vi "CRYSet Statistics Run Flag.vi"(0 "Results in":T1 {"Margin" format="%.2f"}, 1 "Data in":T3 {"Z data" items=["dB", "Lin"]; "X data" items=["dB", "Lin"]; "Y data" items=["dB", "Lin"]; "Z dB ref" format="%.1f"; "Z axis" items=["Log", "Lin"]; "X dB ref" format="%.1f"; "X axis" items=["Log", "Lin"]; "Y axis" items=["Log", "Lin"]; "Y dB ref" format="%.1f"; "Curve"."z" format="%.2f"; "Curve"."y" format="%.2f"; "Curve"."x" format="%.2f"}, 5 "Mode":u16(slide), 9 "Dat_State":bool[](array[boolean]), 11 "Res_state":bool[](array[boolean]), 12 "USL":dbl, 13 "LSL":dbl) -> (4 "Run flag":bool, 10 "Message Numbers":i32[](array[numeric]))   [LabVIEW 2013]
uses:
  Typedef Control/CRYData Cluster Array.ctl
  Typedef Control/CRYData Cluster.ctl
  Typedef Control/CRYResult Cluster Array.ctl
  Typedef Control/CRYResult Cluster.ctl
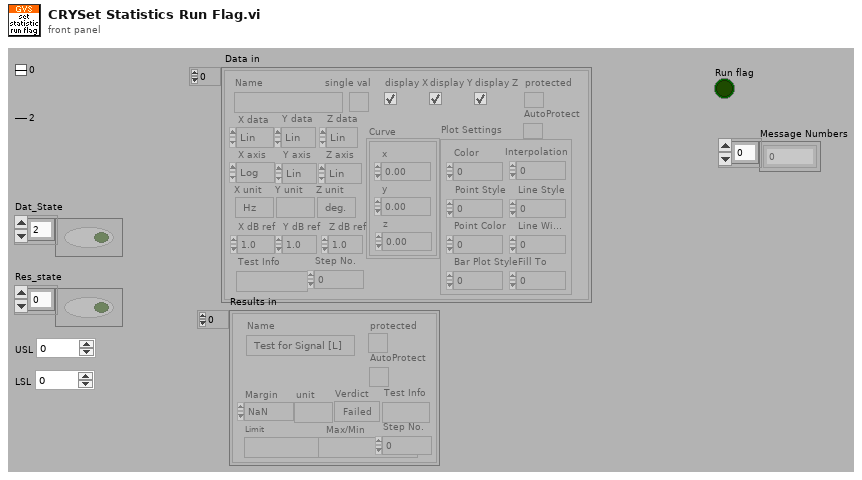
[diagram p1: front panel]
types:
  T1 = typedef "CRYResult Cluster Array.ctl" = T2[]
  T2 = typedef "CRYResult Cluster.ctl" = cluster{"Name":string, "Margin":dbl, "unit":string, "Verdict":bool, "Limit":string, "Max/Min":string, "protected":bool, "Step No.":i32, "Test Info":string, "AutoProtect":bool}
  T3 = typedef "CRYData Cluster Array.ctl" = T4[]
  T4 = typedef "CRYData Cluster.ctl" = cluster{"Name":string, "Curve":cluster{"x":dbl, "y":dbl, "z":dbl}[], "X data":u16, "Y data":u16, "Z data":u16, "X axis":u16, "Y axis":u16, "Z axis":u16, "X unit":string, "Y unit":string, "Z unit":string, "X dB ref":dbl, "Y dB ref":dbl, "Z dB ref":dbl, "single val":bool, "protected":bool, "display X":bool, "display Y":bool, "display Z":bool, "Test Info":string, "Step No.":i32, "Plot Settings":cluster{"Color":u32, "Interpolation":u8, "Point Style":u8, "Line Style":u8, "Point Color":u32, "Line Width":u8, "Bar Plot Style":u8, "Fill To":i16}, "AutoProtect":bool}
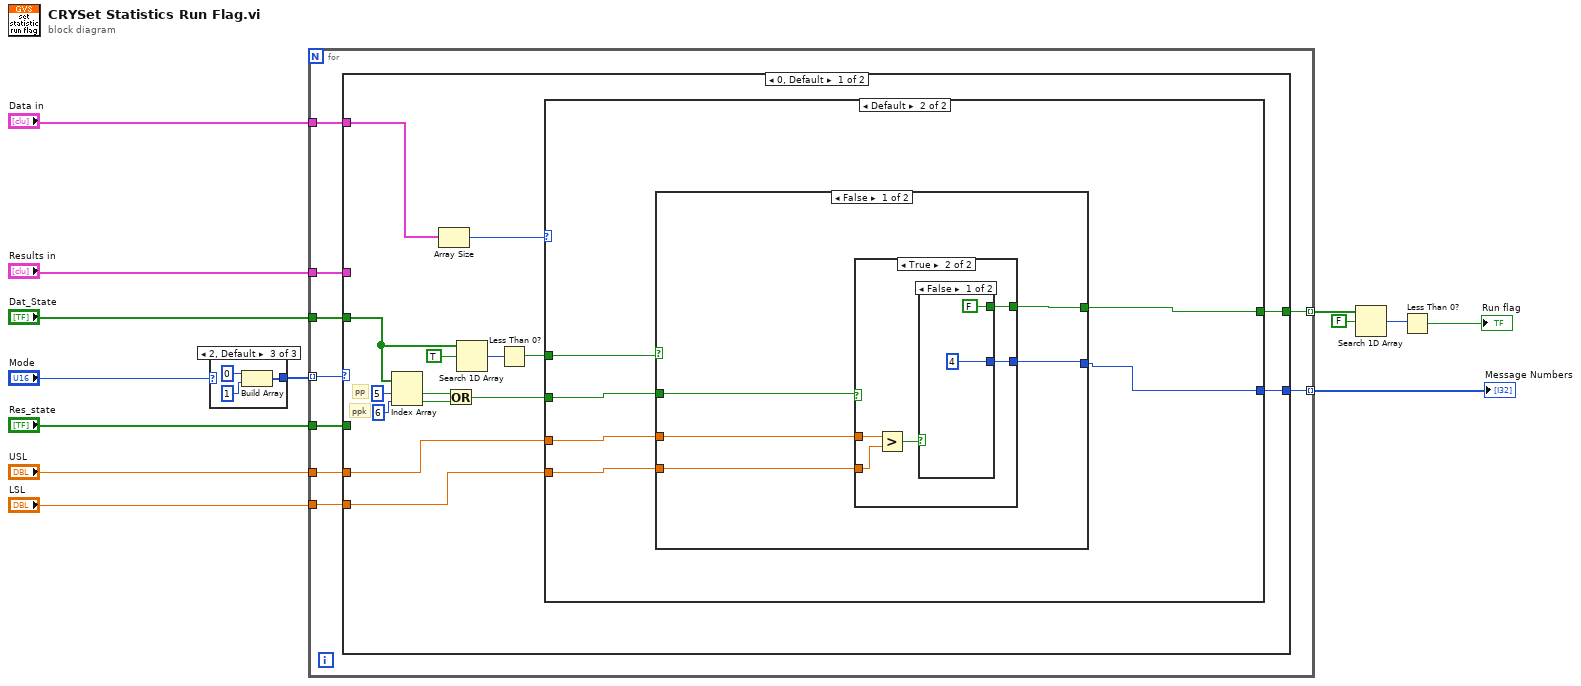
[diagram p0: block diagram]
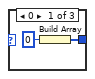
[diagram p2: hidden frame]
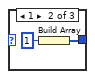
[diagram p3: hidden frame]
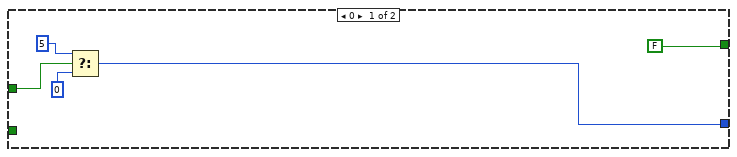
[diagram p4: hidden frame]
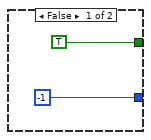
[diagram p5: hidden frame]
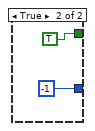
[diagram p6: hidden frame]
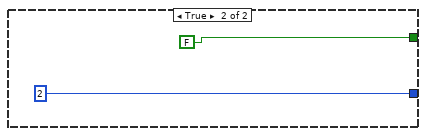
[diagram p7: hidden frame]
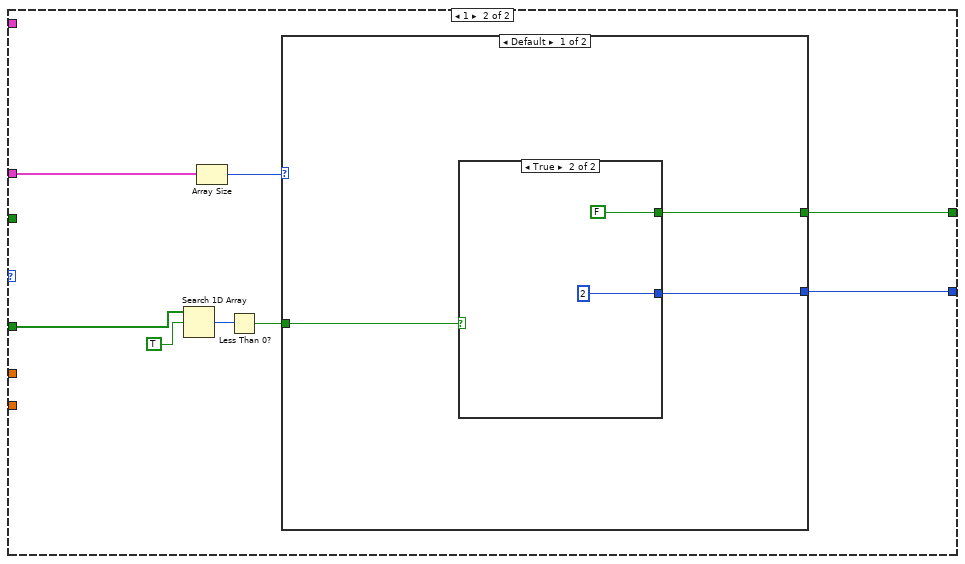
[diagram p8: hidden frame]
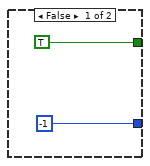
[diagram p9: hidden frame]
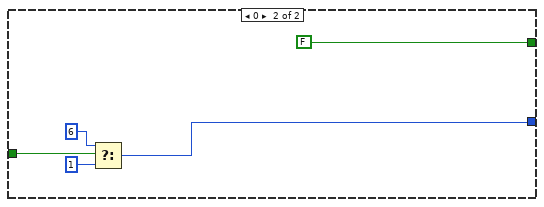
[diagram p10: hidden frame]
diagram:
  n1 = case shown="2, Default" "Mode" {
    tunnel: [w14 w16 w18] -> w6
    frame 0 {
      n2 = Build Array(0 ("No.Ranked(WF)")) -> (w14:i32[])
    }
    frame 1 {
      n3 = Build Array(1 ("No.Ranked(WF)")) -> (w16:i32[])
    }
    frame 2, Default {
      n4 = Build Array(0 ("No.Ranked(WF)"), 1 ("No.Ranked(WF)")) -> (w18:i32[])
    }
  }
  n5 = for {
    tunnel: "Res_state" -> [w29]
    tunnel: "Dat_State" -> [w28]
    tunnel: "USL" -> [w27]
    tunnel: "LSL" -> [w26]
    tunnel: "Data in" -> [w25]
    tunnel: "Results in" -> [w24]
    tunnel: w6 -> [w23] mode=indexing
    tunnel: [w22] -> w5 mode=indexing
    tunnel: [w21] -> w4 mode=indexing
    n6 = case shown="0, Default" w23 {
      tunnel: w29 -> [_ w75]
      tunnel: w28 -> [w34 _]
      tunnel: [w44 w76] -> w22
      tunnel: w25 -> [w40 _]
      tunnel: w27 -> [w42 _]
      tunnel: w26 -> [w41 _]
      tunnel: w24 -> [_ w80]
      tunnel: [w30 w74] -> w21
      frame 0, Default {
        # "ppk"
        # "pp"
        n7 = Index Array(array=w34, index #1=5 ("index"), index #2=6 ("index")) -> (element #1=w33:bool, element #2=w32:bool)
        n8 = Array Size(array=w40) -> (size(s)=w37:i32)
        n9 = Or(x=w33, y=w32) -> (x .or. y?=w31:bool)
        n10 = Search 1D Array(1D array=w34, element=TRUE) -> (index of element=w39:i32)  [unwired: 1 out]
        n11 = Less Than 0?(x=w39) -> (x < 0?=w38:bool)
        n12 = case shown="Default" w37 {
          tunnel: [w46 w54] -> w44
          tunnel: w38 -> [w49 w55]
          tunnel: w42 -> [_ w52]
          tunnel: w41 -> [_ w51]
          tunnel: w31 -> [_ w53]
          tunnel: [FALSE ("Run flag") w50] -> w30
          frame 0 {
            n13 = Select(t=5, s=w49, f=0) -> (s? t:f=w46:i32)
          }
          frame Default {
            n14 = case shown="False" w55 {
              tunnel: [w59 2] -> w54
              tunnel: w53 -> [w60 _]
              tunnel: w52 -> [w58 _]
              tunnel: w51 -> [w57 _]
              tunnel: [w56 FALSE ("Run flag")] -> w50
              frame False {
                n15 = case shown="True" w60 {
                  tunnel: [-1 w64] -> w59
                  tunnel: w58 -> [_ w67]
                  tunnel: w57 -> [_ w66]
                  tunnel: [TRUE ("Run flag") w63] -> w56
                  frame False {
                  }
                  frame True {
                    n16 = Greater?(x=w67, y=w66) -> (0:w65:bool)
                    n17 = case shown="False" w65 {
                      tunnel: [4 -1] -> w64
                      tunnel: [FALSE ("Run flag") TRUE ("Run flag")] -> w63
                      frame False {
                      }
                      frame True {
                      }
                    }
                  }
                }
              }
              frame True {
              }
            }
          }
        }
      }
      frame 1 {
        n18 = Search 1D Array(1D array=w75, element=TRUE) -> (index of element=w78:i32)  [unwired: 1 out]
        n19 = Array Size(array=w80) -> (size(s)=w79:i32)
        n20 = Less Than 0?(x=w78) -> (x < 0?=w77:bool)
        n21 = case shown="Default" w79 {
          tunnel: w77 -> [w84 w93]
          tunnel: [w83 w90] -> w76
          tunnel: [w82 FALSE ("Run flag")] -> w74
          frame Default {
            n22 = case shown="True" w84 {
              tunnel: [-1 ("f") 2 ("f")] -> w83
              tunnel: [TRUE ("Run flag") FALSE ("Run flag")] -> w82
              frame False {
              }
              frame True {
              }
            }
          }
          frame 0 {
            n23 = Select(t=6, s=w93, f=1) -> (s? t:f=w90:i32)
          }
        }
      }
    }
  }
  "Message Numbers" <- w5
  n24 = Search 1D Array(1D array=w4, element=FALSE) -> (index of element=w2:i32)  [unwired: 1 in]
  n25 = Less Than 0?(x=w2) -> (x < 0?=→"Run flag":bool)
